vi "Start Cyclic Data Query.vi"(8 "error in (no error)":errorcluster, 10 "Query Period (ms)":i32=1000, 11 "Sensor in":refnum<class "Sensor.lvclass">) -> (0 "error out":errorcluster, 3 "Sensor out":refnum<class "Sensor.lvclass">)   [LabVIEW 2020, in "Sensor.lvlib" / "Sensor.lvclass"]
uses:
  Sensor.lvclass
  C:/Program Files (x86)/National Instruments/LabVIEW 2020/vi.lib/ActorFramework/Actor/Actor.lvclass
  Sensor Messages/Data Query Msg/Data Query Msg.lvclass
  C:/Program Files (x86)/National Instruments/LabVIEW 2020/vi.lib/ActorFramework/Message/Message.lvclass
  <vilib>/ActorFramework/Message Enqueuer/Message Priority.ctl
  Sensor.lvclass/Sensor.ctl
  <vilib>/ActorFramework/Actor/Actor.lvclass/Actor.ctl
  <vilib>/ActorFramework/Message Enqueuer/Message Enqueuer.lvclass/Message Enqueuer.ctl
  <vilib>/ActorFramework/Message Enqueuer/Init from Existing Queue.vi
  <vilib>/ActorFramework/Message Enqueuer/Message Enqueuer.lvclass
  <vilib>/ActorFramework/Actor/Actor.lvclass
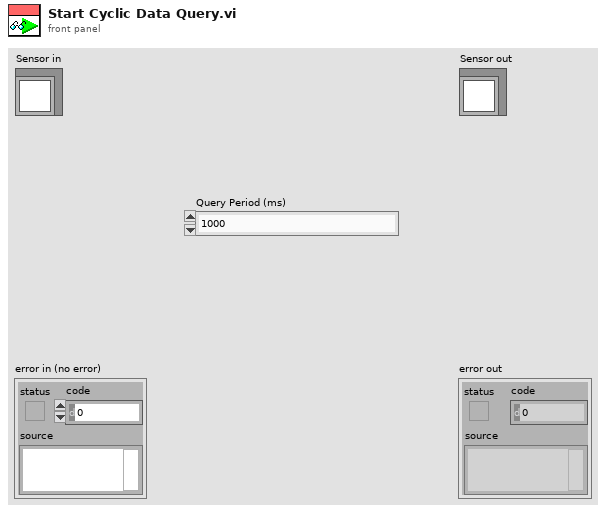
[diagram p1: front panel]
types:
  T1 = typedef "Actor Framework.lvlib/Message Enqueuer.lvclass/Message Priority.ctl" = enum16{"Low", "Normal", "High"}
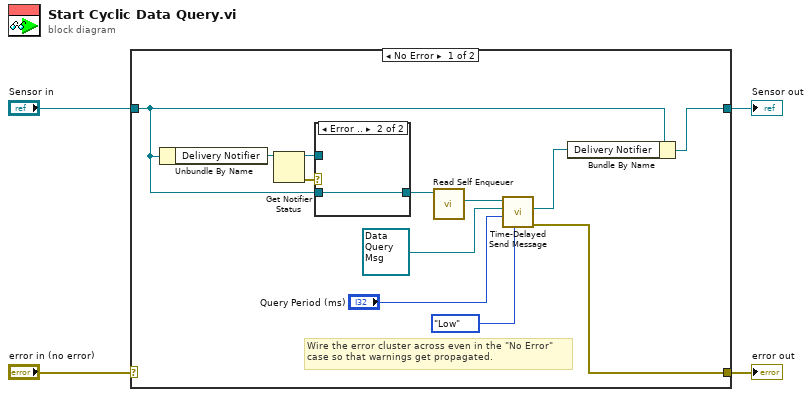
[diagram p0: block diagram]
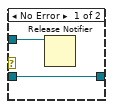
[diagram p2: hidden frame]
diagram:
  n1 = case shown="No Error" "error in (no error)" {
    selector: "error in (no error)" -> [_ w21]
    tunnel: [w10 w21] -> w3
    tunnel: [w16 w20] -> w1
    tunnel: "Sensor in" -> [w7 w20]
    frame No Error {
      # "Wire the error cluster across even in the \"No Error\"\ncase so that warnings get propagated."
      n2 = Unbundle By Name(w7) -> ("Delivery Notifier"=w14:refnum<notifier>)
      n3 = Get Notifier Status(notifier=w14) -> (notifier out=w12:refnum<notifier>, error out=w13:errorcluster)  [unwired: 1 in, 3 out]
      n4 = case shown="Error .." w13 {
        tunnel: w12 -> [w18 _]
        tunnel: [w17 w19] -> w8
        tunnel: w7 -> [w17 w19]
        frame No Error {
          n5 = Release Notifier(notifier=w18) -> ()  [unwired: 2 in, 3 out]
        }
        frame Error {
        }
      }
      n6 = call <vilib>:"Read Self Enqueuer.vi"("Actor"=w8) -> ("Self Enqueuer"=w9:refnum<class "Message Enqueuer.lvclass">)  [unwired: 10 in]
      n7 = call <vilib>:"Time-Delayed Send Message.vi"("Message Priority (Normal)"=Message_Priority."Low", "Milliseconds To Wait"="Query Period (ms)", "Message"=refnum<class "Data Query Msg.lvclass"> refnum ("Sensor.lvlib:Data Query Msg.lvclass"), "Message Enqueuer"=w9) -> ("error out"=w10:errorcluster, "Delivery Notifier"=w11:refnum<notifier>)  [unwired: 6 in]
      n8 = Bundle By Name(cluster=w7, "Delivery Notifier"=w11) -> (w16:refnum<class "Sensor.lvclass">)
    }
    frame Error {
    }
  }
  "error out" <- w3
  "Sensor out" <- w1
